vi "Keithley24XX_SR830_LakeShore336_4Probe_Resistance_Measurement_FAST.vi"() -> ()   [LabVIEW 2020]
uses:
  LabVIEW 2020/instr.lib/Lake Shore 336/Public/Data/Sensor Data (Single Reading).vi
  LabVIEW 2020/instr.lib/Stanford Research 830/Public/Data/Read (All Parameters).vi
  LabVIEW 2020/instr.lib/Keithley 24XX/Public/Data/Read (Single Point).vi
  LabVIEW 2020/instr.lib/Keithley 24XX/Keithley 24XX.lvlib
  LabVIEW 2020/instr.lib/Stanford Research 830/Stanford Research 830.lvlib
  LabVIEW 2020/instr.lib/Lake Shore 336/Lake Shore 336.lvlib
panel:
  out "Gate\nVoltage":sgl
  out "Status":sgl
  out "Leakage \nCurrent":sgl
  in  "Temp Vs Time":enum32{"XY Graph", "Waveform (Time)"}(tab)
  out "Temp vs Time : XYGraph":cluster{"Y":dbl[], "Y":dbl[]}[](graph)
  out "Temp vs Time : TimeGraph":cluster{i32, "Sensor Data":dbl}[](graph)
  in  "Data Source (0:Kelvin)":u16(ring) items=["Kelvin", "Celsius", "Sensor Units"]
  in  "Input (0:A)":u16(ring) items=["A", "B", "C", "D"]
  in  "Serial Configuration 2":T1={"Baud Rate"=57600, "Parity"=1, "Data Bits"=7, "Stop Bits"=10, "Flow Control"=0} {"Flow Control" items=["None", "XON/XOFF", "RTS/CTS", "XON/XOFF & RTS/CTS", "DTR/DSR", "XON/XOFF & DTR/DSR"]; "Stop Bits" items=["1.0"=10, "1.5"=15, "2.0"=20]; "Data Bits" items=["7"=7, "8"=8]; "Parity" items=["None", "Odd", "Even", "Mark", "Space"]; "Baud Rate" items=["300"=300, "600"=600, "1200"=1200, "2400"=2400, "4800"=4800, "9600"=9600, "19200"=19200, "38400"=38400, "57600"=57600]}
  in  "LakeShore 336 esource name":refnum<visa-resource-name>="GPIB0::12::INSTR"
  out "dup path":path
  in  "<File Name>.txt (Don't add extension)":string
  in  "Data Save Path:":path=path "C:/Users/labpc/Documents/ProbeStation Users Data"
  in  "I_leak vs Vg":enum32{"XY Graph", "Waveform (Time)"}(tab)
  out "I_leak vs Vg : XYGraph":cluster{"Y":dbl[], "Y":dbl[]}[](graph)
  out "I_leak vs Vg : TimeGraph":cluster{dbl, "Current":sgl}[](graph)
  in  "Gate Voltage\nInitial (V)":dbl
  out "Gate Voltage\nTraversal Direction":enum16{"Upward", "Downward"}(ring)
  in  "Series Resistance \n(Apparatus Constant)":dbl=10000000.0
  in  "stop":bool
  out "Max/Min(-) \nGate Voltage (V)":dbl=80.0
  in  "Gate Voltage \nStep Size (V)":dbl=0.1
  in  "High Gate \nVoltage (V)":dbl
  in  "Low Gate \nVoltage (V)":dbl
  out "Compliance\n Level (A)":dbl=0.1
  in  "Theta vs Vg":enum32{"XY Graph", "Waveform (Time)"}(tab)
  out "Theta vs Vg : XYGraph":cluster{"Y":dbl[], "Y":dbl[]}[](graph)
  out "Theta vs Vg : TimeGraph":cluster{dbl, "Theta-Value":dbl}[](graph)
  in  "R vs Vg":enum32{"XY Graph", "Waveform (Time)"}(tab)
  out "Resistance vs Vg : XYGraph":cluster{"Y":dbl[], "Y":dbl[]}[](graph)
  out "R vs Vg : TimeGraph":cluster{dbl, dbl}[](graph)
  in  "Sensitivity (Initial Value)":i16(ring)=17 items=["Auto Gain"=-1, "2 nV/fA"=0, "5 nV/fA"=1, "10 nV/fA"=2, "20 nV/fA"=3, "50 nV/fA"=4, "100 nV/fA"=5, "200 nV/fA"=6, "500 nV/fA"=7, "1 uV/pA"=8, "2 uV/pA"=9, "5 uV/pA"=10, "10 uV/pA"=11, "20 uV/pA"=12, "50 uV/pA"=13, "100 uV/pA"=14, "200 uV/pA"=15, "500 uV/pA"=16, "1 mV/nA"=17, "2 mV/nA"=18, "5 mV/nA"=19, "10 mV/nA"=20, "20 mV/nA"=21, "50 mV/nA"=22, "100 mV/nA"=23, "200 mV/nA"=24, "500 mV/mA"=25, "1 V/uA"=26]
  in  "Dynamic Reserve (-1 = Auto)":i16(ring)=-1 items=["Auto Reserve"=-1, "High Reserve"=0, "Normal"=1, "Low Noise"=2]
  in  "Input Connection (0: Single-Ended Voltage)":u16(ring)=1 items=["Single-Ended Voltage", "Differential Voltage", "1 MOhm Current Gain", "100 MOhm Current Gain"]
  out "Input Coupling (0: AC)":u16(ring) items=["AC", "DC"]
  in  "Time Constant (8: 100ms)":u16(ring)=9 items=["10 us", "30 us", "100 us", "300 us", "1 ms", "3 ms", "10 ms", "30 ms", "100 ms", "300 ms", "1 s", "3 s", "10 s", "30 s", "100 s", "300 s", "1 ks", "3 ks", "10 ks", "30 ks"]
  in  "SR830 VISA resource name":refnum<visa-resource-name>="GPIB0::10::INSTR"
  in  "Trigger Source (0: Internal)":u16(ring) items=["Internal", "External"]
  out "Manual Phase (0 Degree)":dbl
  out "Detection Harmonic Number":dbl=1.0
  out "External Reference Trigger (0: Sine Zero Crossing)":u16(ring) items=["Sine Zero Crossing", "TTL Rising Edge", "TTL Falling Edge"]
  in  "Internal Reference Frequency (1000 Hz)":dbl=17.0
  in  "Reference Source (1: Internal)":u16(ring)=1 items=["External", "Internal"]
  in  "Sine Output Amplitude (V)":dbl=1.0
  in  "Serial Configuration":T1={"Baud Rate"=9600, "Parity"=0, "Data Bits"=8, "Stop Bits"=10, "Flow Control"=0} {"Flow Control" items=["None", "XON/XOFF", "RTS/CTS", "XON/XOFF & RTS/CTS", "DTR/DSR", "XON/XOFF & DTR/DSR"]; "Stop Bits" items=["1.0"=10, "1.5"=15, "2.0"=20]; "Data Bits" items=["7"=7, "8"=8]; "Parity" items=["None", "Odd", "Even", "Mark", "Space"]; "Baud Rate" items=["300"=300, "600"=600, "1200"=1200, "2400"=2400, "4800"=4800, "9600"=9600, "19200"=19200]}
  in  "Keithley24XX VISA resource name":refnum<visa-resource-name>="GPIB0::21::INSTR" caption="Keithley 24XX VISA resource name"
  out "Interal Measurement Time":u32
  # "Lake Shore 336 Temp Contr."
  # "SR830 Lock In Amplifier"
  # "MAKE SURE THE SOURCE METER IS ON TO ENSURE NO UNINTENDED JUMPS. PROGRAM WILL KEEP SOURCE METER ON ONCE RUN."
  # "Keithley 2400 SourceMeter"
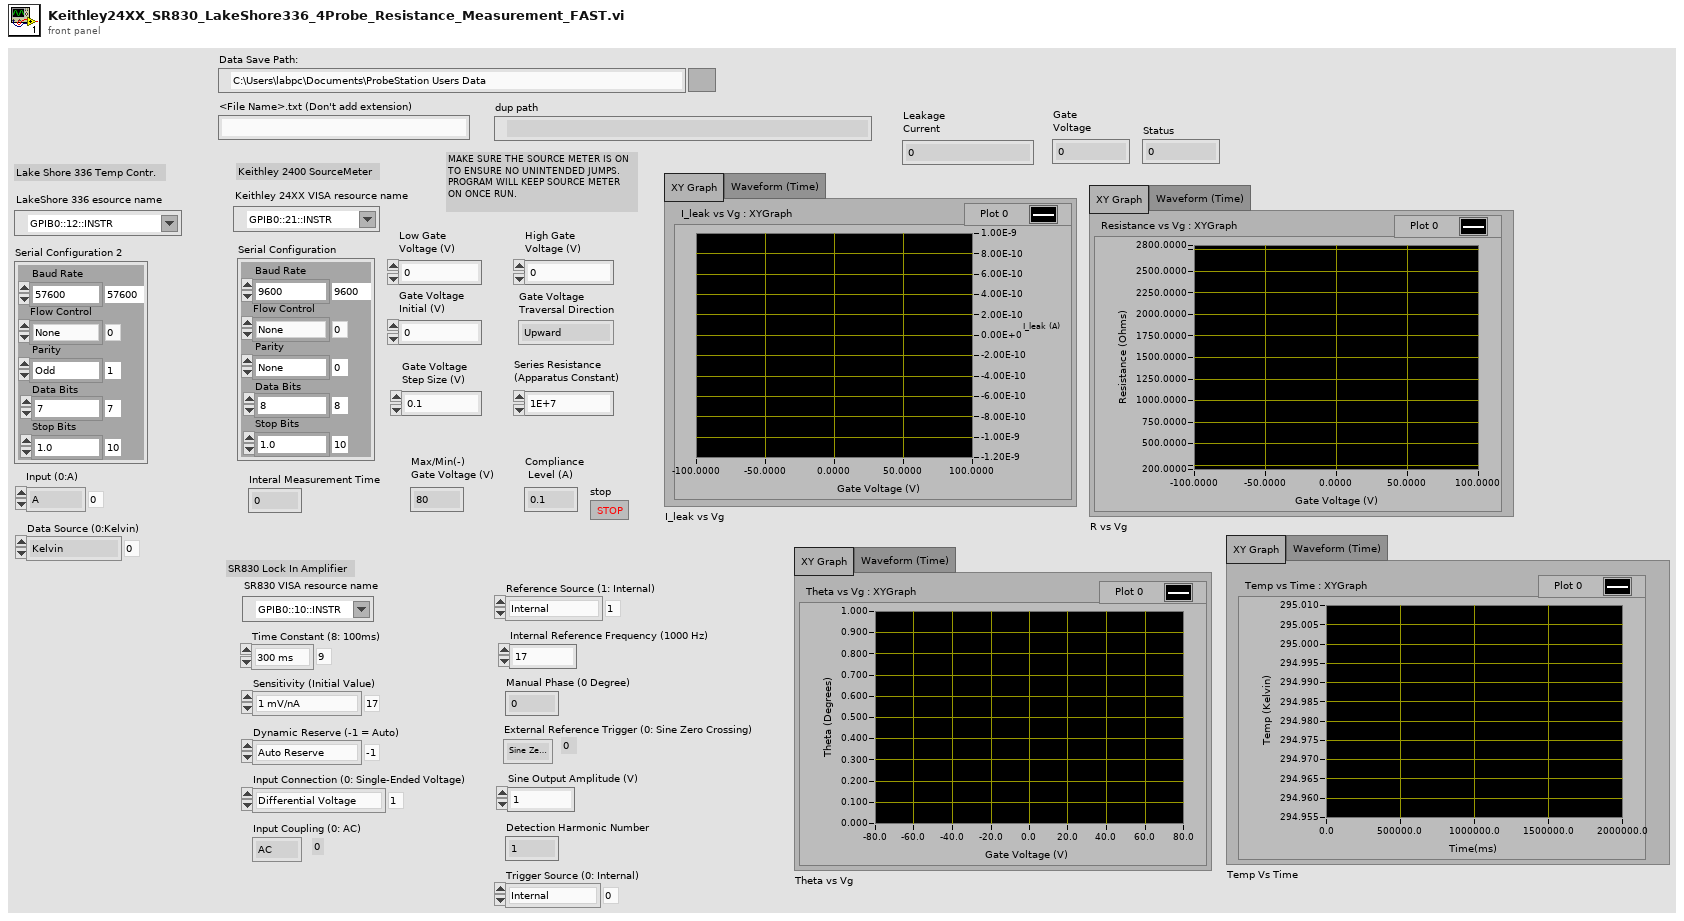
[diagram p1: front panel]
types:
  T1 = cluster{"Baud Rate":u32, "Parity":u16, "Data Bits":u16, "Stop Bits":u16, "Flow Control":u16}
  T2 = enum16{"open", "replace", "create", "open or create", "replace or create", "replace or create with confirmation"}
  T3 = cluster{"X-Value":dbl, "Y-Value":dbl, "R-Value":dbl, "Theta-Value":dbl, "Aux In 1 Value":dbl, "Aux In 2 Value":dbl, "Aux In 3 Value":dbl, "Aux In 4 Value":dbl, "Reference Frequency":dbl, "Channel 1 Display":dbl, "Channel 2 Display":dbl}
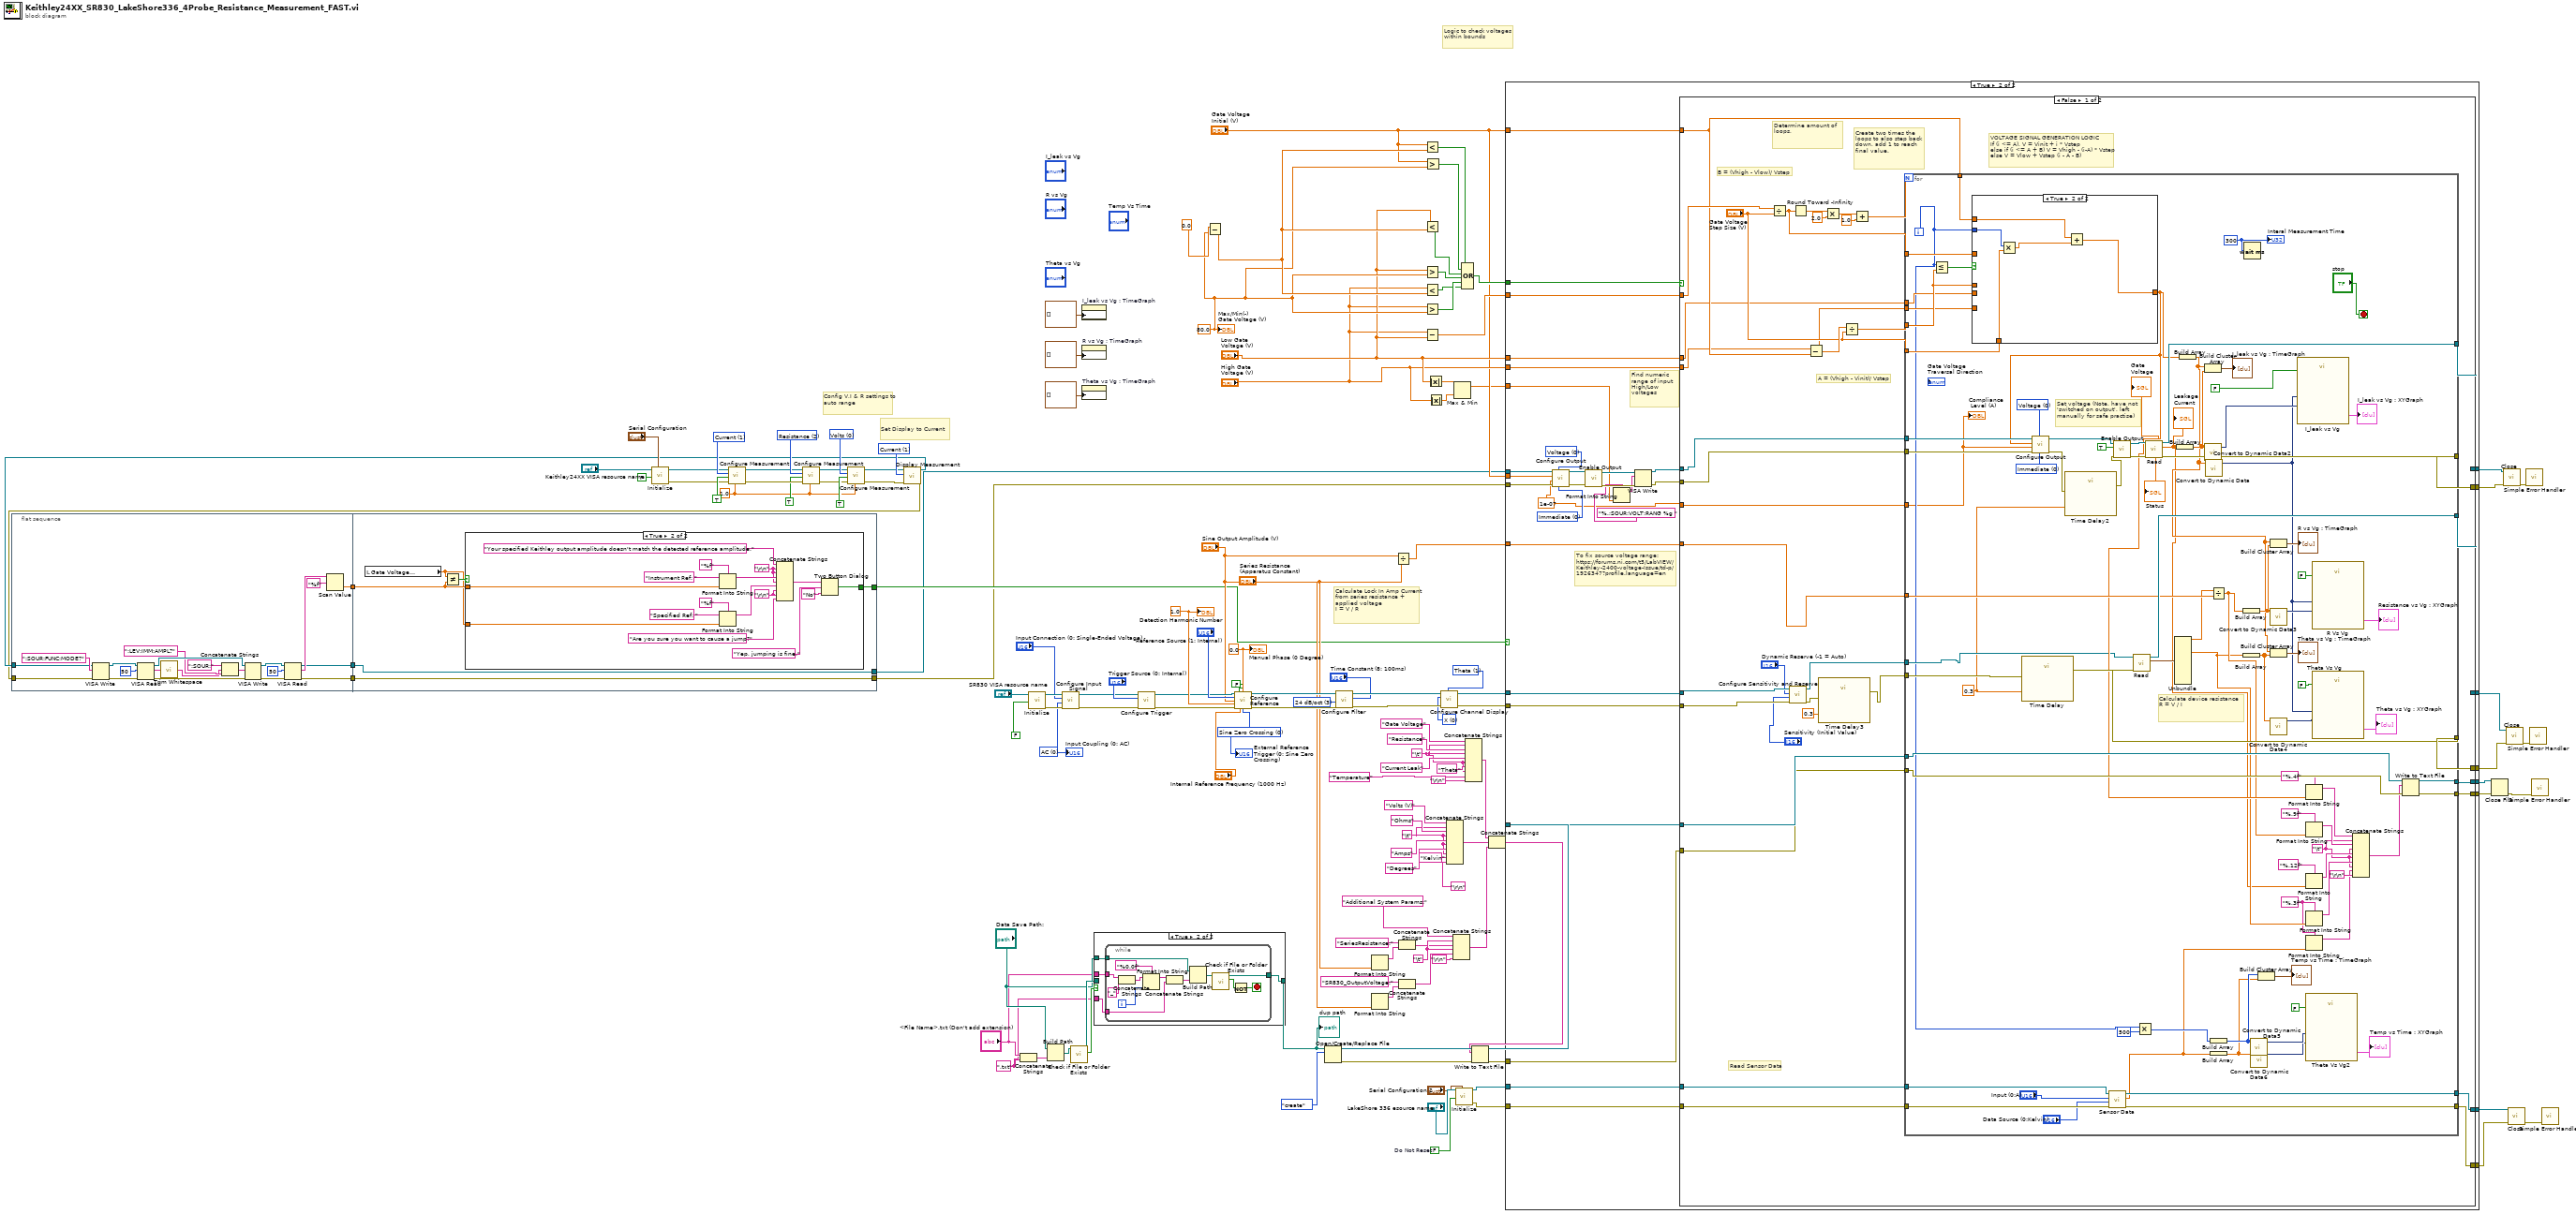
[diagram p0: block diagram]
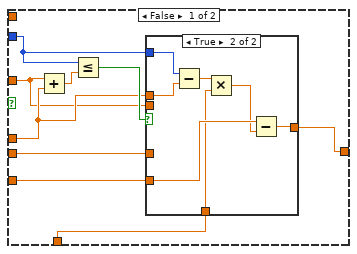
[diagram p3: hidden frame]
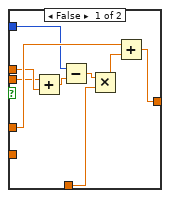
[diagram p4: hidden frame]
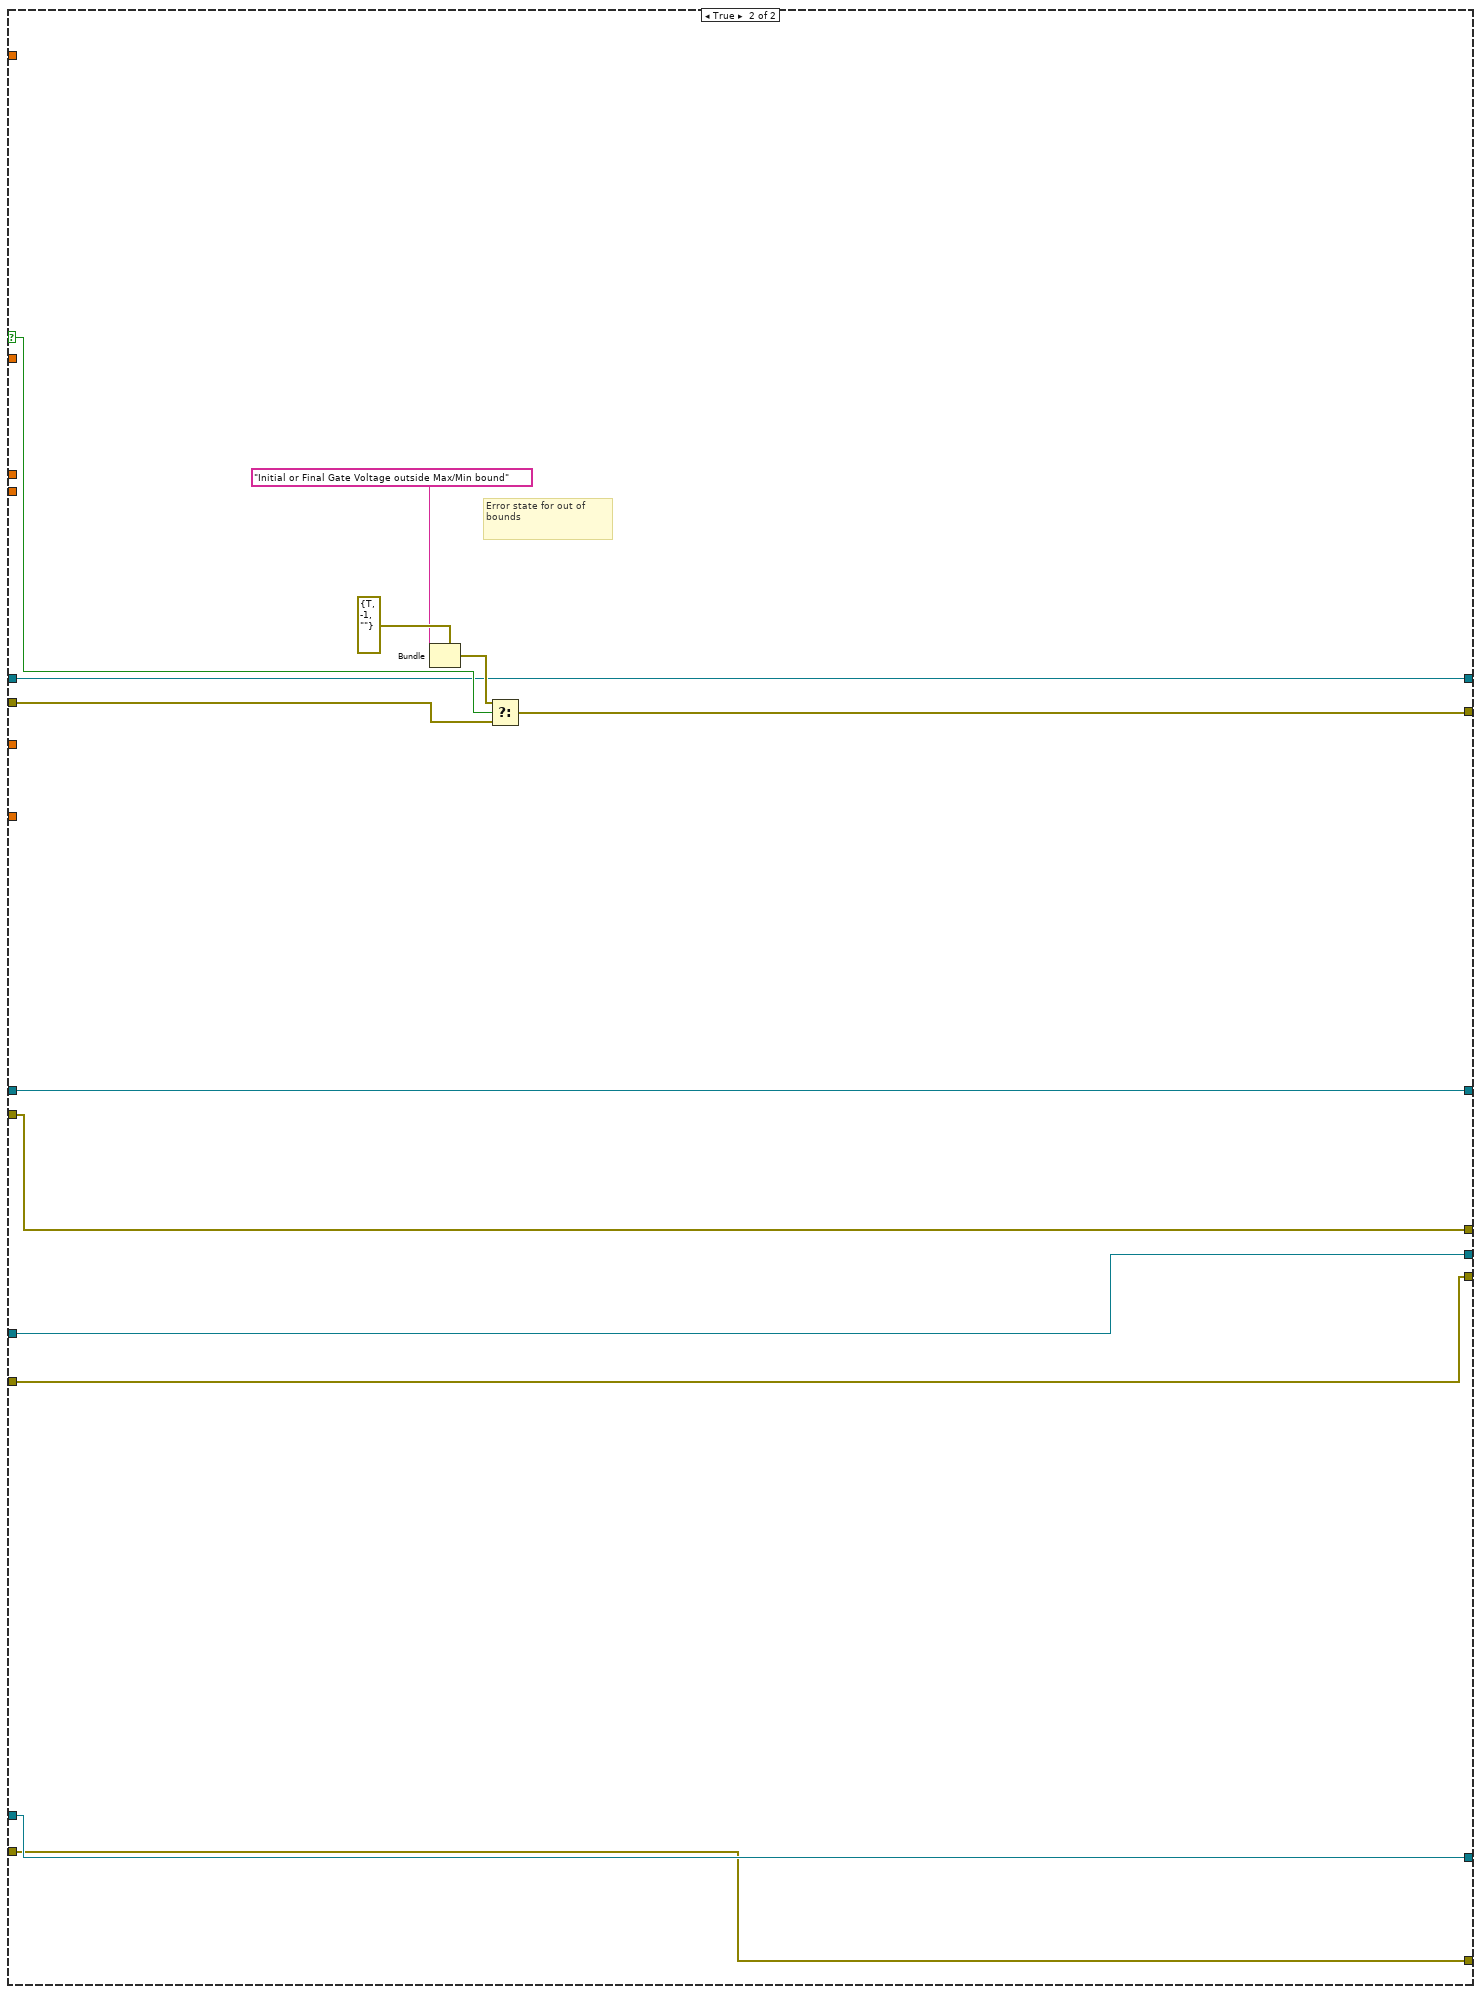
[diagram p5: hidden frame]
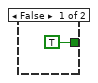
[diagram p6: hidden frame]
diagram:
  w1 = u16 3 items=["6 dB/oct", "12 dB/oct", "18 db/oct", "24 dB/oct"] ("Low Pass Filter Slope (1: 12dB/oct)")
  w28 = FALSE  # Do Not Reset
  w34 = "\t"
  w17 = "\t"
  w19 = "\t"
  w62 = ".txt"
  w69 = 1.0 ("Manual Range (1.0)")
  w93 = 0.0 ("Manual Phase (0 Degree)")
  w94 = 1.0 ("Detection Harmonic Number (1)")
  w95 = u16 0 items=["Sine Zero Crossing", "TTL Rising Edge", "TTL Falling Edge"] ("External Reference Trigger (0: Sine Zero Crossing)")
  w99 = u16 0 items=["AC", "DC"] ("Input Coupling (0: AC)")
  w81 = u16 0 items=["X", "R", "X Noise", "Aux In 1", "Aux In 2"] ("Channel 1 Display (0: X)")
  w109 = u16 1 items=["Y", "Theta", "Y Noise", "Aux In 3", "Aux In 4"] ("Channel 2 Display  (0: Y)")
  w114 = u16 1 items=["Voltage", "Current", "Resistance"] ("Displayed Measurement (0: Voltage)")
  w123 = u16 2 items=["Volts", "Current", "Resistance"] ("Function (0: Volts)")
  w127 = u16 1 items=["Volts", "Current", "Resistance"] ("Function (0: Volts)")
  w70 = 80.0
  w133 = u16 0 items=["Volts", "Current", "Resistance"] ("Function (0: Volts)")
  # "Logic to check voltages within bounds"
  # "Calculate Lock In Amp Current from series resistance + applied voltage\nI = V / R"
  # "Set Display to Current"
  # "Config V,I & R settings to auto range"
  n1 = flat-sequence {
    tunnel: [w137] -> w11
    tunnel: [w138] -> w10
    tunnel: [w139] -> w9
    tunnel: w8 -> [w136]
    tunnel: w7 -> [w135]
    tunnel: w11 -> [w158]
    tunnel: w10 -> [w157]
    tunnel: w9 -> [w161]
    tunnel: [w158] -> w3
    tunnel: [w157] -> w5
    tunnel: [w156] -> w6
    frame #0 {
      n2 = VISA Write(VISA resource name=w136, write buffer=":SOUR:FUNC:MODE?", error in (no error)=w135) -> (VISA resource name out=w152:refnum<visa-resource-name>, error out=w155:errorcluster)  [unwired: 1 out]
      n3 = VISA Read(VISA resource name=w152, byte count=u32 50, error in (no error)=w155) -> (VISA resource name out=w147:refnum<visa-resource-name>, read buffer=w141:string, error out=w148:errorcluster)  [unwired: 1 out]
      n4 = call <vilib>:"Trim Whitespace.vi"("string"=w141) -> ("trimmed string"=w140:string)  [unwired: 1 in]
      n5 = Concatenate Strings(":SOUR:" ("string"), w140, ":LEV:IMM:AMPL?" ("string")) -> (w144:string)
      n6 = VISA Write(VISA resource name=w147, write buffer=w144, error in (no error)=w148) -> (VISA resource name out=w149:refnum<visa-resource-name>, error out=w151:errorcluster)  [unwired: 1 out]
      n7 = VISA Read(VISA resource name=w149, byte count=u32 50, error in (no error)=w151) -> (VISA resource name out=w137:refnum<visa-resource-name>, read buffer=w142:string, error out=w138:errorcluster)  [unwired: 1 out]
      n8 = Scan Value(string=w142, format string="%f") -> (value=w139:dbl)  [unwired: 1 in, 1 out]
    }
    frame #1 {
      n9 = local read "Gate Voltage\nInitial (V)"() -> (w159:dbl)
      n10 = Not Equal?(x=w159, y=w161) -> (x != y?=w160:bool)
      n11 = case shown="True" w160 {
        tunnel: [TRUE ("T button?") w169] -> w156
        tunnel: w161 -> [_ w164]
        tunnel: w159 -> [_ w163]
        frame False {
        }
        frame True {
          w167 = "\r\n"
          w165 = "\r\n"
          n12 = Format Into String(format string="%f", initial string="Instrument Ref: ", w164) -> (resulting string=w171:string)  [unwired: 1 in, 1 out]
          n13 = Format Into String(format string="%f", initial string="Specified Ref: ", w163) -> (resulting string=w170:string)  [unwired: 1 in, 1 out]
          n14 = Concatenate Strings("Your specified Keithley output amplitude doesn't match the detected reference amplitude." ("message"), w165, w165, w171, w165, w170, w167, w167, "Are you sure you want to cause a jump?" ("string")) -> (w176:string)
          n15 = Two Button Dialog(message=w176, 1:"No" ("F button name (\"Cancel\")"), 2:"Yep, jumping is fine." ("T button name (\"OK\")")) -> (T button?=w169:bool)
        }
      }
    }
  }
  n16 = call "Initialize.vi"("Serial Configuration"="Serial Configuration", "Reset (True)"=FALSE, "VISA resource name"="Keithley24XX VISA resource name") -> ("error out"=w118:errorcluster, "VISA resource name out"=w119:refnum<visa-resource-name>)  [unwired: 7 in]
  n17 = call "Configure Measurement.vi"("Manual Range (1.0)"=w69, "error in (no error)"=w118, "Enable Auto Range (T:Enable)"=TRUE, "Function (0: Volts)"=w127, "VISA resource name"=w119) -> ("error out"=w125:errorcluster, "VISA resource name out"=w120:refnum<visa-resource-name>)  [unwired: 5 in]
  n18 = call "Configure Measurement.vi"("Manual Range (1.0)"=w69, "error in (no error)"=w125, "Enable Auto Range (T:Enable)"=TRUE, "Function (0: Volts)"=w123, "VISA resource name"=w120) -> ("error out"=w122:errorcluster, "VISA resource name out"=w121:refnum<visa-resource-name>)  [unwired: 5 in]
  n19 = call "Configure Measurement.vi"("Manual Range (1.0)"=w69, "error in (no error)"=w122, "Enable Auto Range (T:Enable)"=TRUE, "Function (0: Volts)"=w133, "VISA resource name"=w121) -> ("error out"=w112:errorcluster, "VISA resource name out"=w113:refnum<visa-resource-name>)  [unwired: 5 in]
  n20 = call "Display Measurement.vi"("error in (no error)"=w112, "Displayed Measurement (0: Voltage)"=w114, "VISA resource name"=w113) -> ("error out"=w7:errorcluster, "VISA resource name out"=w8:refnum<visa-resource-name>)  [unwired: 7 in]
  n21 = Concatenate Strings("<File Name>.txt (Don't add extension)", w62) -> (w68:string)
  n22 = call "Initialize.vi"("Reset (True)"=FALSE, "VISA resource name"="SR830 VISA resource name") -> ("error out"=w106:errorcluster, "VISA resource name out"=w107:refnum<visa-resource-name>)  [unwired: 8 in]
  n23 = Build Path(base path="Data Save Path:", name or relative path=w68) -> (appended path=w67:path)
  n24 = call "Configure Input Signal.vi"("error in (no error)"=w106, "Input Coupling (0: AC)"=w99, "Input Connection (0: Single-Ended Voltage)"="Input Connection (0: Single-Ended Voltage)", "VISA resource name"=w107) -> ("error out"=w90:errorcluster, "VISA resource name out"=w91:refnum<visa-resource-name>)  [unwired: 6 in]
  n25 = call <vilib>:"Check if File or Folder Exists.vi"("path"=w67) -> ("file or folder exists?"=w66:bool, "dup path"=w65:path)  [unwired: 8 in, 1 out]
  n26 = property on="I_leak vs Vg : TimeGraph" class="WFChart (strict)"("History Data"=cluster{dbl, "Current":sgl}[] []) -> ()  [unwired: 2 in, 2 out]
  n27 = property on="R vs Vg : TimeGraph" class="WFChart (strict)"("History Data"=cluster{dbl, dbl}[] []) -> ()  [unwired: 2 in, 2 out]
  n28 = property on="Theta vs Vg : TimeGraph" class="WFChart (strict)"("History Data"=cluster{dbl, "Theta-Value":dbl}[] []) -> ()  [unwired: 2 in, 2 out]
  n29 = case shown="True" w66 {
    tunnel: [w179 w180] -> w59
    tunnel: w65 -> [w179 _]
    tunnel: "Data Save Path:" -> [_ w181]
    tunnel: "<File Name>.txt (Don't add extension)" -> [_ w183]
    tunnel: w62 -> [_ w182]
    frame False {
    }
    frame True {
      n30 = while {
        tunnel: w183 -> [w186]
        tunnel: w182 -> [w191]
        tunnel: w181 -> [w189]
        tunnel: [w187] -> w180
        i -> [w193]
        stop <- w195 stop-if-true
        n31 = Concatenate Strings(w186, "_" ("string")) -> (w185:string)
        n32 = Format Into String(format string="%0.0f", initial string=w185, w193) -> (resulting string=w192:string)  [unwired: 1 in, 1 out]
        n33 = Concatenate Strings(w192, w191) -> (w190:string)
        n34 = Build Path(base path=w189, name or relative path=w190) -> (appended path=w188:path)
        n35 = call <vilib>:"Check if File or Folder Exists.vi"("path"=w188) -> ("file or folder exists?"=w196:bool, "dup path"=w187:path)  [unwired: 8 in, 1 out]
        n36 = Not(x=w196) -> (.not. x?=w195:bool)
      }
    }
  }
  "dup path" <- w59
  n37 = call "Configure Trigger.vi"("error in (no error)"=w90, "Trigger Source (0: Internal)"="Trigger Source (0: Internal)", "VISA resource name"=w91) -> ("error out"=w88:errorcluster, "VISA resource name out"=w89:refnum<visa-resource-name>)  [unwired: 7 in]
  n38 = Subtract(x=0.0, y=w70) -> (x-y=w75:dbl)
  n39 = call "Configure Reference.vi"("VISA resource name"=w89, "Auto Phase (T: Enabled)"=FALSE, "Manual Phase (0 Degree)"=w93, "Reference Source (1: Internal)"="Reference Source (1: Internal)", "Sine Output Amplitude (1 V)"="Sine Output Amplitude (V)", "Detection Harmonic Number (1)"=w94, "error in (no error)"=w88, "Internal Reference Frequency (1000 Hz)"="Internal Reference Frequency (1000 Hz)", "External Reference Trigger (0: Sine Zero Crossing)"=w95) -> ("VISA resource name out"=w96:refnum<visa-resource-name>, "error out"=w97:errorcluster)  [unwired: 5 in]
  n40 = Open/Create/Replace File(file path (use dialog)=w59, operation (0:open)=T2."create") -> (refnum out=w60:refnum<file>, error out=w58:errorcluster)  [unwired: 4 in, 1 out]
  n41 = call "Configure Filter.vi"("error in (no error)"=w97, "Low Pass Filter Slope (1: 12dB/oct)"=w1, "Time Constant (8: 100ms)"="Time Constant (8: 100ms)", "VISA resource name"=w96) -> ("error out"=w116:errorcluster, "VISA resource name out"=w115:refnum<visa-resource-name>)  [unwired: 6 in]
  n42 = Format Into String("Series Resistance \n(Apparatus Constant)") -> (resulting string=w52:string)  [unwired: 3 in, 1 out]
  n43 = Format Into String("Sine Output Amplitude (V)") -> (resulting string=w51:string)  [unwired: 3 in, 1 out]
  n44 = Divide(x="Sine Output Amplitude (V)", y="Series Resistance \n(Apparatus Constant)") -> (x/y=w87:dbl)
  n45 = Concatenate Strings("SeriesResistance:" ("string"), w52) -> (w33:string)
  n46 = Concatenate Strings("SR830_OutputVoltage:" ("string"), w51) -> (w32:string)
  n47 = Less?(x="Gate Voltage\nInitial (V)", y=w75) -> (x < y?=w73:bool)
  n48 = Less?(x="Low Gate \nVoltage (V)", y=w75) -> (x < y?=w79:bool)
  n49 = Greater?(x="Low Gate \nVoltage (V)", y=w70) -> (0:w78:bool)
  n50 = Less?(x="High Gate \nVoltage (V)", y=w75) -> (x < y?=w76:bool)
  n51 = Greater?(x="High Gate \nVoltage (V)", y=w70) -> (0:w77:bool)
  n52 = Subtract(x="High Gate \nVoltage (V)", y="Low Gate \nVoltage (V)") -> (x-y=w71:dbl)
  n53 = Greater?(x="Gate Voltage\nInitial (V)", y=w70) -> (0:w74:bool)
  n54 = Absolute Value(x="Low Gate \nVoltage (V)") -> (abs(x)=w15:dbl)
  n55 = Absolute Value(x="High Gate \nVoltage (V)") -> (abs(x)=w14:dbl)
  n56 = call "Configure Channel Display.vi"("Channel 2 Display  (0: Y)"=w109, "error in (no error)"=w116, "Channel 1 Display (0: X)"=w81, "VISA resource name"=w115) -> ("error out"=w104:errorcluster, "VISA resource name out"=w105:refnum<visa-resource-name>)  [unwired: 6 in]
  n57 = Concatenate Strings("Volts (V)" ("string"), w17, "Ohms" ("string"), w17, "Amps" ("string"), w17, "Degrees" ("string"), w17, "Kelvin" ("string"), "\r\n") -> (w45:string)
  n58 = Concatenate Strings("Additional System Params:" ("string"), w34, w33, w34, w32, "\r\n") -> (w35:string)
  n59 = Max & Min(x=w15, y=w14) -> (max(x,y)=w2:dbl)  [unwired: 1 out]
  n60 = call "Initialize.vi"("Serial Configuration"="Serial Configuration 2", "Reset (True)"=w28, "VISA resource name"="LakeShore 336 esource name") -> ("error out"=w23:errorcluster, "VISA resource name out"=w22:refnum<visa-resource-name>)  [unwired: 7 in]
  n61 = Compound Arithmetic op=OR(w73, w74, w79, w78, w77, w76) -> (w72:bool)
  n62 = Concatenate Strings("Gate Voltage" ("string"), w19, "Resistance" ("string"), w19, "Current Leak" ("string"), w19, "Theta" ("string"), w19, "Temperature" ("string"), "\r\n") -> (w46:string)
  n63 = Concatenate Strings(w46, w45, w35) -> (w30:string)
  n64 = Write to Text File(file (use dialog)=w60, text=w30, error in=w58) -> (refnum out=w56:refnum<file>, error out=w55:errorcluster)  [unwired: 1 in, 1 out]
  n65 = case shown="True" w6 {
    tunnel: [w204 w239] -> w131
    tunnel: [w203 w238] -> w130
    tunnel: w105 -> [w202 w237]
    tunnel: w104 -> [w201 w236]
    tunnel: [w202 w235] -> w103
    tunnel: [w201 w234] -> w102
    tunnel: w87 -> [_ w233]
    tunnel: w72 -> [_ w232]
    tunnel: w71 -> [_ w231]
    tunnel: w56 -> [w200 w230]
    tunnel: w55 -> [w199 w229]
    tunnel: [w200 w228] -> w54
    tunnel: [w199 w227] -> w53
    tunnel: [w197 w226] -> w25
    tunnel: [w198 w225] -> w24
    tunnel: w23 -> [w197 w224]
    tunnel: w22 -> [w198 w223]
    tunnel: "Low Gate \nVoltage (V)" -> [_ w222]
    tunnel: "High Gate \nVoltage (V)" -> [_ w221]
    tunnel: "Gate Voltage\nInitial (V)" -> [_ w220]
    tunnel: w5 -> [w203 w212]
    tunnel: "Gate Voltage\nInitial (V)" -> [_ w211]
    tunnel: w3 -> [w204 w210]
    tunnel: w2 -> [_ w208]
    frame False {
    }
    frame True {
      w214 = u16 0 items=["Immediate", "Triggered"] ("Output Type  (0: Immediate)")
      w207 = 1e-07 ("Compliance  Level (0.1)")
      w213 = u16 0 items=["Voltage", "Current"] ("Source Mode  (0: Voltage)")
      # "Find numeric range of input High/Low voltages"
      # "To fix source voltage range:\nhttps://forums.ni.com/t5/LabVIEW/Keithley-2400-voltage-Issue/td-p/1926347?profile.language=en"
      n66 = call "Configure Output.vi"("Output Type  (0: Immediate)"=w214, "Source Mode  (0: Voltage)"=w213, "error in (no error)"=w212, "Compliance  Level (0.1)"=w207, "Output Level (0)"=w211, "VISA resource name"=w210) -> ("error out"=w219:errorcluster, "VISA resource name out"=w218:refnum<visa-resource-name>)  [unwired: 4 in]
      n67 = call "Enable Output.vi"("error in (no error)"=w219, "VISA resource name"=w218) -> ("error out"=w217:errorcluster, "VISA resource name out"=w216:refnum<visa-resource-name>)  [unwired: 8 in]
      n68 = Format Into String(format string="%.;SOUR:VOLT:RANG %g ", w208) -> (resulting string=w215:string)  [unwired: 2 in, 1 out]
      n69 = VISA Write(VISA resource name=w216, write buffer=w215, error in (no error)=w217) -> (VISA resource name out=w205:refnum<visa-resource-name>, error out=w206:errorcluster)  [unwired: 1 out]
      n70 = case shown="False" w232 {
        selector: w232 -> [_ w406]
        tunnel: w206 -> [w276 w405]
        tunnel: w205 -> [w241 w400]
        tunnel: [w275 w400] -> w239
        tunnel: [w274 w401] -> w238
        tunnel: w237 -> [w269 w399]
        tunnel: w236 -> [w270 w398]
        tunnel: [w272 w399] -> w235
        tunnel: [w271 w398] -> w234
        tunnel: w233 -> [w266 _]
        tunnel: w231 -> [w261 _]
        tunnel: w222 -> [w254 _]
        tunnel: w221 -> [w255 _]
        tunnel: w220 -> [w257 _]
        tunnel: w230 -> [w250 w397]
        tunnel: w229 -> [w249 w396]
        tunnel: [w248 w397] -> w228
        tunnel: [w247 w396] -> w227
        tunnel: [w243 w394] -> w226
        tunnel: [w242 w395] -> w225
        tunnel: w224 -> [w245 w394]
        tunnel: w223 -> [w244 w395]
        tunnel: w207 -> [w240 _]
        frame False {
          # "Read Sensor Data"
          # "VOLTAGE SIGNAL GENERATION LOGIC\nIf (i <= A), V = Vinit + i * Vstep\nelse if (i <= A + B) V = Vhigh - (i-A) * Vstep\nelse V = Vlow + Vstep (i - A - B)"
          # "B = (Vhigh - Vlow)/ Vstep"
          # "A = (Vhigh - Vinit)/ Vstep"
          # "Create two times the loops to also step back down, add 1 to reach final value."
          # "Determine amount of loops,"
          n71 = Divide(x=w261, y="Gate Voltage \nStep Size (V)") -> (x/y=w256:dbl)
          n72 = call "Configure Sensitivity and Reserve.vi"("error in (no error)"=w270, "Sensitivity (-1: Auto gain)"="Sensitivity (Initial Value)", "Dynamic Reserve (-1: Auto Reserve)"="Dynamic Reserve (-1 = Auto)", "VISA resource name"=w269) -> ("error out"=w252:errorcluster, "VISA resource name out"=w268:refnum<visa-resource-name>)  [unwired: 6 in]
          n73 = Round Toward -Infinity(1:w256) -> (0:w264:dbl)
          n74 = Subtract(x=w255, y=w257) -> (x-y=w260:dbl)
          n75 = call "Time Delay3"("error in (no error)"=w252, "Delay Time (s)"=0.3) -> ("error out"=w253:errorcluster)  [unwired: 9 in]
          n76 = Multiply(x=w264, y=2.0) -> (x*y=w263:dbl)
          n77 = Divide(x=w260, y="Gate Voltage \nStep Size (V)") -> (x/y=w258:dbl)
          n78 = Add(x=w263, y=1.0) -> (x+y=w262:dbl)
          n79 = for {
            N: w262 -> [_]
            tunnel: w241 -> [w359]
            tunnel: w276 -> [w324]
            tunnel: [w363] -> w275
            tunnel: [w362] -> w274
            tunnel: [w352] -> w272
            tunnel: [w353] -> w271
            tunnel: w268 -> [w305]
            tunnel: w253 -> [w306]
            tunnel: w266 -> [w350]
            tunnel: "Gate Voltage \nStep Size (V)" -> [w330]
            tunnel: w258 -> [w328]
            tunnel: w257 -> [w331]
            tunnel: w256 -> [w329]
            tunnel: w255 -> [w327]
            tunnel: w254 -> [w326]
            tunnel: w250 -> [w321]
            tunnel: w249 -> [w320]
            tunnel: [w319] -> w248
            tunnel: [w318] -> w247
            tunnel: w245 -> [w297]
            tunnel: w244 -> [w296]
            tunnel: [w295] -> w243
            tunnel: [w294] -> w242
            tunnel: w240 -> [w277]
            i -> [w288]
            stop <- "stop" stop-if-true
            w285 = "%.3f" ("format string")
            w282 = "\t"
            w325 = u16 0 items=["Immediate", "Triggered"] ("Output Type  (0: Immediate)")
            w304 = 0.3 ("Delay Time (s)")
            w360 = u32 300 ("milliseconds to wait")
            w355 = u16 0 items=["Voltage", "Current"] ("Source Mode  (0: Voltage)")
            # "Calculate device resistance\nR = V / I"
            # "Set voltage (Note, have not 'switched on output', left manually for safe practise)"
            n80 = Less Or Equal?(x=w288, y=w328) -> (x <= y?=w332:bool)
            n81 = case shown="True" w332 {
              tunnel: [w370 w389] -> w312
              tunnel: w331 -> [_ w392]
              tunnel: w288 -> [w367 w393]
              tunnel: w330 -> [w368 w390]
              tunnel: w329 -> [w364 _]
              tunnel: w328 -> [w366 _]
              tunnel: w327 -> [w369 _]
              tunnel: w326 -> [w365 _]
              frame False {
                n82 = Add(x=w364, y=w366) -> (x+y=w371:dbl)
                n83 = Less Or Equal?(x=w367, y=w371) -> (x <= y?=w372:bool)
                n84 = case shown="True" w372 {
                  tunnel: [w378 w387] -> w370
                  tunnel: w369 -> [_ w388]
                  tunnel: w368 -> [w380 w385]
                  tunnel: w367 -> [w375 w384]
                  tunnel: w366 -> [w374 w383]
                  tunnel: w365 -> [w381 _]
                  tunnel: w364 -> [w373 _]
                  frame False {
                    n85 = Add(x=w373, y=w374) -> (x+y=w376:dbl)
                    n86 = Subtract(x=w375, y=w376) -> (x-y=w377:dbl)
                    n87 = Multiply(x=w377, y=w380) -> (x*y=w379:dbl)
                    n88 = Add(x=w381, y=w379) -> (x+y=w378:dbl)
                  }
                  frame True {
                    n89 = Subtract(x=w384, y=w383) -> (x-y=w386:dbl)
                    n90 = Multiply(x=w386, y=w385) -> (x*y=w382:dbl)
                    n91 = Subtract(x=w388, y=w382) -> (x-y=w387:dbl)
                  }
                }
              }
              frame True {
                n92 = Multiply(x=w393, y=w390) -> (x*y=w391:dbl)
                n93 = Add(x=w392, y=w391) -> (x+y=w389:dbl)
              }
            }
            n94 = call "Time Delay"("error in (no error)"=w306, "Delay Time (s)"=w304) -> ("error out"=w348:errorcluster)  [unwired: 9 in]
            n95 = call "Configure Output.vi"("Output Type  (0: Immediate)"=w325, "Source Mode  (0: Voltage)"=w355, "error in (no error)"=w324, "Compliance  Level (0.1)"=w277, "Output Level (0)"=w312, "VISA resource name"=w359) -> ("error out"=w323:errorcluster, "VISA resource name out"=w358:refnum<visa-resource-name>)  [unwired: 4 in]
            n96 = call "Time Delay2"("error in (no error)"=w323, "Delay Time (s)"=w304) -> ("error out"=w322:errorcluster)  [unwired: 9 in]
            n97 = call-poly "Sensor Data.vi"("error in (no error)"=w297, "Data Source (0:Kelvin)"="Data Source (0:Kelvin)", "Input (0:A)"="Input (0:A)", "VISA resource name"=w296) -> ("error out"=w295:errorcluster, "Sensor Data"=w284:dbl, "VISA resource name out"=w294:refnum<visa-resource-name>)  [unwired: 5 in]
            n98 = call "Enable Output.vi"("error in (no error)"=w322, "Enable Output (T: Enable)"=TRUE, "VISA resource name"=w358) -> ("error out"=w357:errorcluster, "VISA resource name out"=w356:refnum<visa-resource-name>)  [unwired: 7 in]
            n99 = call-poly "Read.vi"("error in (no error)"=w348, "VISA resource name"=w305) -> ("error out"=w353:errorcluster, "Parameter Values"=w351:T3, "VISA resource name out"=w352:refnum<visa-resource-name>)  [unwired: 7 in]
            n100 = Multiply(x=w288, y=500) -> (x*y=w286:i32)
            n101 = call-poly "Read.vi"("VISA resource name"=w356, "error in (no error)"=w357) -> ("Voltage"=→"Gate\nVoltage":sgl, "VISA resource name out"=w363:refnum<visa-resource-name>, "Current"=w280:sgl, "Status"=→"Status":sgl, "error out"=w362:errorcluster)  [unwired: 7 in, 2 out]
            "Leakage \nCurrent" <- w280
            n102 = Unbundle(w351) -> ("X-Value"=w349:dbl, "Theta-Value"=w310:dbl)  [unwired: 9 out]
            n103 = Build Array(w280) -> (w345:sgl[])
            n104 = Build Array(w312) -> (w301:dbl[])
            n105 = Build Cluster Array(w301, w345) -> (→"I_leak vs Vg : TimeGraph":cluster{dbl, "Current":sgl}[])
            n106 = call "Convert to Dynamic Data2"("Array"=w345) -> ("Dynamic Data Type"=w344:dynamicdata)  [unwired: 3 in]
            n107 = call "Convert to Dynamic Data"("Array"=w301) -> ("Dynamic Data Type"=w300:dynamicdata)  [unwired: 3 in]
            n108 = Build Array(w286) -> (w298:i32[])
            n109 = Build Array(w284) -> (w290:dbl[])
            n110 = Divide(x=w349, y=w350) -> (x/y=w311:dbl)
            n111 = Build Array(w311) -> (w343:dbl[])
            n112 = Build Array(w310) -> (w341:dbl[])
            n113 = Wait (ms)(milliseconds to wait=w360) -> ()  [unwired: 1 out]
            n114 = call "Convert to Dynamic Data5"("Array"=w298) -> ("Dynamic Data Type"=w299:dynamicdata)  [unwired: 3 in]
            n115 = call "Convert to Dynamic Data6"("Array"=w290) -> ("Dynamic Data Type"=w291:dynamicdata)  [unwired: 3 in]
            n116 = Build Cluster Array(w298, w290) -> (→"Temp vs Time : TimeGraph":cluster{i32, "Sensor Data":dbl}[])
            n117 = Build Cluster Array(w301, w343) -> (→"R vs Vg : TimeGraph":cluster{dbl, dbl}[])
            n118 = call "Convert to Dynamic Data3"("Array"=w343) -> ("Dynamic Data Type"=w342:dynamicdata)  [unwired: 3 in]
            n119 = Build Cluster Array(w301, w341) -> (→"Theta vs Vg : TimeGraph":cluster{dbl, "Theta-Value":dbl}[])
            n120 = call "Convert to Dynamic Data4"("Array"=w341) -> ("Dynamic Data Type"=w340:dynamicdata)  [unwired: 3 in]
            n121 = call "I_leak vs Vg"("Reset"=FALSE, "Y Input"=w344, "X Input"=w300) -> ("XY Graph"=→"I_leak vs Vg : XYGraph":cluster{"X":dbl[], "Y":dbl[]}[])  [unwired: 7 in, 1 out]
            n122 = Format Into String(format string="%.4f", w312) -> (resulting string=w317:string)  [unwired: 2 in, 1 out]
            n123 = Format Into String(format string="%.9f", w311) -> (resulting string=w316:string)  [unwired: 2 in, 1 out]
            n124 = Format Into String(format string="%.12f", w280) -> (resulting string=w315:string)  [unwired: 2 in, 1 out]
            n125 = Format Into String(format string=w285, w310) -> (resulting string=w314:string)  [unwired: 2 in, 1 out]
            n126 = Format Into String(format string=w285, w284) -> (resulting string=w281:string)  [unwired: 2 in, 1 out]
            n127 = call "Theta Vs Vg2"("Reset"=FALSE, "Y Input"=w291, "X Input"=w299) -> ("XY Graph"=→"Temp vs Time : XYGraph":cluster{"X":dbl[], "Y":dbl[]}[])  [unwired: 7 in, 1 out]
            n128 = call "R Vs Vg"("Reset"=FALSE, "Y Input"=w342, "X Input"=w300) -> ("XY Graph"=→"Resistance vs Vg : XYGraph":cluster{"X":dbl[], "Y":dbl[]}[])  [unwired: 7 in, 1 out]
            n129 = call "Theta Vs Vg"("Reset"=FALSE, "Y Input"=w340, "X Input"=w300) -> ("XY Graph"=→"Theta vs Vg : XYGraph":cluster{"X":dbl[], "Y":dbl[]}[])  [unwired: 7 in, 1 out]
            n130 = Concatenate Strings(w317, w282, w316, w282, w315, w282, w314, w282, w281, "\r\n") -> (w313:string)
            n131 = Write to Text File(file (use dialog)=w321, text=w313, error in=w320) -> (refnum out=w319:refnum<file>, error out=w318:errorcluster)  [unwired: 1 in, 1 out]
            "Compliance\n Level (A)" <- w277
            "Interal Measurement Time" <- w360
          }
        }
        frame True {
          # "Error state for out of bounds"
          n132 = Bundle(cluster=errorcluster {"status"=TRUE, "code"=-1, "source"=""} ("error constant"), "source"="Initial or Final Gate Voltage outside Max/Min bound") -> (w402:errorcluster)  [unwired: 2 in]
          n133 = Select(t=w402, s=w406, f=w405) -> (s? t:f=w401:errorcluster)
        }
      }
    }
  }
  n134 = Close File(refnum=w54, error in=w53) -> (error out=w57:errorcluster)  [unwired: 1 out]
  n135 = call "Close.vi"("error in (no error)"=w130, "VISA resource name"=w131) -> ("error out"=w129:errorcluster)  [unwired: 9 in]
  n136 = call "Close.vi"("error in (no error)"=w102, "VISA resource name"=w103) -> ("error out"=w117:errorcluster)  [unwired: 9 in]
  n137 = call "Close.vi"("error in (no error)"=w25, "VISA resource name"=w24) -> ("error out"=w26:errorcluster)  [unwired: 9 in]
  n138 = call <vilib>:"Simple Error Handler.vi"("error in (no error)"=w129) -> ()  [unwired: 4 in, 5 out]
  n139 = call <vilib>:"Simple Error Handler.vi"("error in (no error)"=w117) -> ()  [unwired: 4 in, 5 out]
  n140 = call <vilib>:"Simple Error Handler.vi"("error in (no error)"=w57) -> ()  [unwired: 4 in, 5 out]
  n141 = call <vilib>:"Simple Error Handler.vi"("error in (no error)"=w26) -> ()  [unwired: 4 in, 5 out]
  "Max/Min(-) \nGate Voltage (V)" <- w70
  "Input Coupling (0: AC)" <- w99
  "External Reference Trigger (0: Sine Zero Crossing)" <- w95
  "Detection Harmonic Number" <- w94
  "Manual Phase (0 Degree)" <- w93
